vi "LocateAndDistance.vi"(4 "BlobDataR In":dbl[][](array[numeric]), 5 "ImageR In":T1, 6 "BlobDataL In":dbl[][](array[numeric]), 7 "ImageL In":T1) -> (0 "Dist":cluster{"Distance":dbl, "Area":dbl}[](array[cluster]), 1 "ImageR Out":T1, 2 "Distance":T2(array[cluster]), 3 "ImageL Out":T1)   [LabVIEW 2011]
uses:
  <vilib>/vision/Image Controls.llb/IMAQ Image.ctl
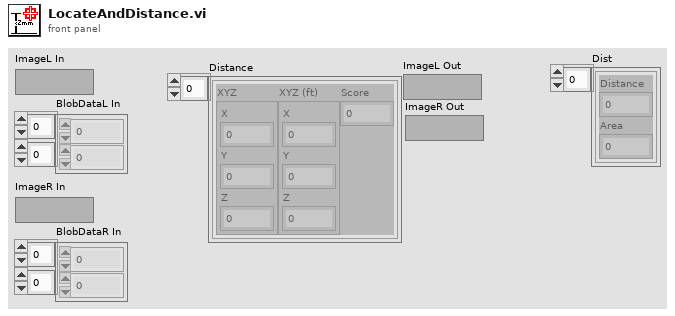
[diagram p1: front panel]
types:
  T1 = typedef "IMAQ Image.ctl" = refnum<image>
  T2 = cluster{"XYZ":cluster{"X":dbl, "Y":dbl, "Z":dbl}, "XYZ (ft)":cluster{"X":dbl, "Y":dbl, "Z":dbl}, "Score":dbl}[]
  T3 = cluster{cluster{"BlobData In[0]":dbl, "BlobData In[1]":dbl}, cluster{"BlobData In[2]":dbl, "BlobData In[3]":dbl}, cluster{"BlobData In[4]":dbl, "BlobData In[5]":dbl, "BlobData In[6]":dbl, "BlobData In[7]":dbl}, cluster{"BlobData In[8]":dbl, "BlobData In[9]":dbl}, "BlobData In[10]":dbl}[]
  T4 = cluster{cluster{cluster{"BlobData In[0]":dbl, "BlobData In[1]":dbl}, cluster{"BlobData In[2]":dbl, "BlobData In[3]":dbl}, cluster{"BlobData In[4]":dbl, "BlobData In[5]":dbl, "BlobData In[6]":dbl, "BlobData In[7]":dbl}, cluster{"BlobData In[8]":dbl, "BlobData In[9]":dbl}, "BlobData In[10]":dbl}, cluster{cluster{"BlobData In[0]":dbl, "BlobData In[1]":dbl}, cluster{"BlobData In[2]":dbl, "BlobData In[3]":dbl}, cluster{"BlobData In[4]":dbl, "BlobData In[5]":dbl, "BlobData In[6]":dbl, "BlobData In[7]":dbl}, cluster{"BlobData In[8]":dbl, "BlobData In[9]":dbl}, "BlobData In[10]":dbl}, "Score":dbl}[]
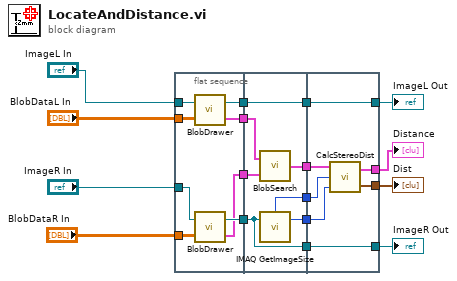
[diagram p0: block diagram]
diagram:
  n1 = flat-sequence {
    tunnel: "ImageL In" -> [w25]
    tunnel: "BlobDataL In" -> [w24]
    tunnel: "ImageR In" -> [w23]
    tunnel: "BlobDataR In" -> [w22]
    tunnel: [w21] -> w13
    tunnel: [w20] -> w12
    tunnel: [w19] -> w11
    tunnel: [w18] -> w10
    tunnel: w13 -> [w27]
    tunnel: w12 -> [w32]
    tunnel: w11 -> [w26]
    tunnel: w10 -> [w31]
    tunnel: [w30] -> w9
    tunnel: [w29] -> w7
    tunnel: [w28] -> w6
    tunnel: [w27] -> w5
    tunnel: [w26] -> w3
    tunnel: w9 -> [w39]
    tunnel: [w34] -> w8
    tunnel: w7 -> [w38]
    tunnel: w6 -> [w37]
    tunnel: [w36] -> w4
    tunnel: w5 -> [w36]
    tunnel: [w35] -> w2
    tunnel: w3 -> [w35]
    tunnel: [w33] -> w1
    frame #0 {
      n2 = call "BlobDrawer.vi"("BlobData In"=w24, "Image In"=w25) -> ("BlobData"=w20:T3, "Image Out"=w21:T1)
      n3 = call "BlobDrawer.vi"("BlobData In"=w22, "Image In"=w23) -> ("BlobData"=w18:T3, "Image Out"=w19:T1)
    }
    frame #1 {
      n4 = call "BlobSearch.vi"("BlobData R"=w31, "BlobData L"=w32) -> ("BlobData"=w30:T4)
      n5 = call "IMAQ GetImageSize"("Image"=w26) -> ("Y Resolution"=w28:i32, "X Resolution"=w29:i32)  [unwired: 3 in, 1 out]
    }
    frame #2 {
      n6 = call "CalcStereoDist.vi"("Image Height"=w37, "Image Width"=w38, "BlobData"=w39) -> ("Dist"=w33:cluster{"Distance":dbl, "Area":dbl}[], "Distance"=w34:T2)
    }
  }
  "Distance" <- w8
  "ImageL Out" <- w4
  "ImageR Out" <- w2
  "Dist" <- w1
